vi "Event--Mouse Down.vi"(8 "error in":errorcluster, 10 "Event Data":T2, 11 "Selector in":refnum<class "Selector.lvclass">) -> (0 "error out":errorcluster, 1 "Enable Change":bool, 2 "Name":string, 3 "Selector out":refnum<class "Selector.lvclass">)   [LabVIEW 2019, in "Selector.lvclass"]
uses:
  Selector.lvclass
  <vilib>/Utility/miscctls.llb/LVPositionTypeDef.ctl
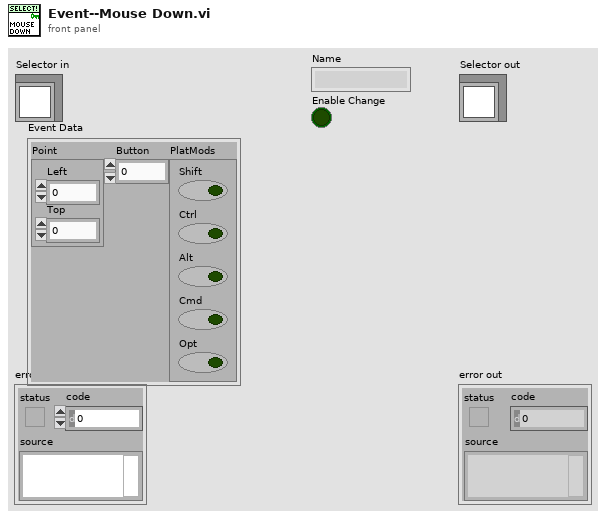
[diagram p1: front panel]
types:
  T1 = typedef "LVPositionTypeDef.ctl" = cluster{"Left":i32, "Top":i32}
  T2 = cluster{"Point":T1, "Button":u16, "PlatMods":cluster{"Shift":bool, "Ctrl":bool, "Alt":bool, "Cmd":bool, "Opt":bool}}
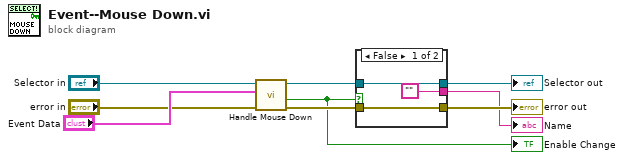
[diagram p0: block diagram]
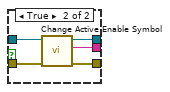
[diagram p2: hidden frame]
diagram:
  n1 = call-dynamic "Handle Mouse Down.vi"("error in (no error)"="error in", "Event Data"="Event Data", "Selector in"="Selector in") -> ("error out"=w3:errorcluster, "Enable Change"=w2:bool, "Selector out"=w4:refnum<class "Selector.lvclass">)  [unwired: 6 in]
  "Enable Change" <- w2
  n2 = case shown="False" w2 {
    tunnel: w4 -> [w12 w17]
    tunnel: w3 -> [w11 w16]
    tunnel: [w11 w15] -> w5
    tunnel: [w12 w14] -> w6
    tunnel: ["" w13] -> w1
    frame False {
    }
    frame True {
      n3 = call "Change Active Enable Symbol.vi"("error in (no error)"=w16, "Selector in"=w17) -> ("error out"=w15:errorcluster, "Name"=w13:string, "Selector out"=w14:refnum<class "Selector.lvclass">)  [unwired: 7 in]
    }
  }
  "error out" <- w5
  "Selector out" <- w6
  "Name" <- w1
